vi "Path String to Path Array.vi"(0 "Path String":string, 11 "error in (no error)":errorcluster) -> (4 "array":string[](array[string]), 15 "error out":errorcluster)   [LabVIEW 2017, in "Advanced Variant Tools.lvlib"]
uses:
  Advanced Variant Tools.lvlib
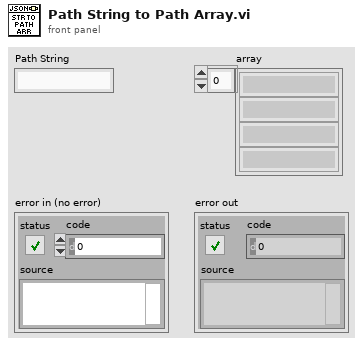
[diagram p1: front panel]
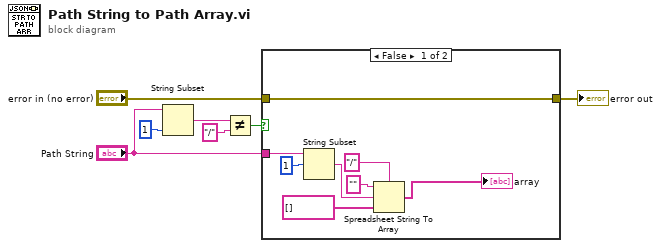
[diagram p0: block diagram]
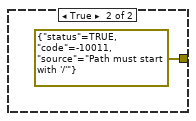
[diagram p2: hidden frame]
diagram:
  n1 = String Subset(string="Path String", length (rest)=1 ("length (rest)")) -> (substring=w5:string)  [unwired: 1 in]
  n2 = Not Equal?(x=w5, y="/") -> (x != y?=w3:bool)
  n3 = case shown="False" w3 {
    tunnel: "Path String" -> [w10 _]
    tunnel: [w11 errorcluster {"status"=TRUE, "code"=-10011, "source"="Path must start with '/'"} ("error constant")] -> w2
    tunnel: "error in (no error)" -> [w11 _]
    frame False {
      n4 = String Subset(string=w10, offset (0)=1) -> (substring=w9:string)  [unwired: 1 in]
      n5 = Spreadsheet String To Array(delimiter (Tab)="/", format string="", spreadsheet string=w9, array type (2D Dbl)=string[] []) -> (array=→"array":string[])
    }
    frame True {
    }
  }
  "error out" <- w2
